vi "flashV4.vi"() -> ()   [LabVIEW 2017]
panel:
  out "error out 2":errorcluster={"status"=TRUE, "code"=56, "source"="UDP Read in UDP.vi->flash.vi"}
  out "error out":errorcluster={"status"=TRUE, "code"=56, "source"="UDP Read in UDP.vi->flash.vi"}
  out "Out 2":u8 format="%.0x"
  out "data out 3":string
  out "data out 2":string
  out "Array":i32[](array[numeric])
  out "String":string
  in  "error in (no error)":errorcluster
  out "Out":u8 format="%.0x"
  in  "address":string="192.168.10.23"
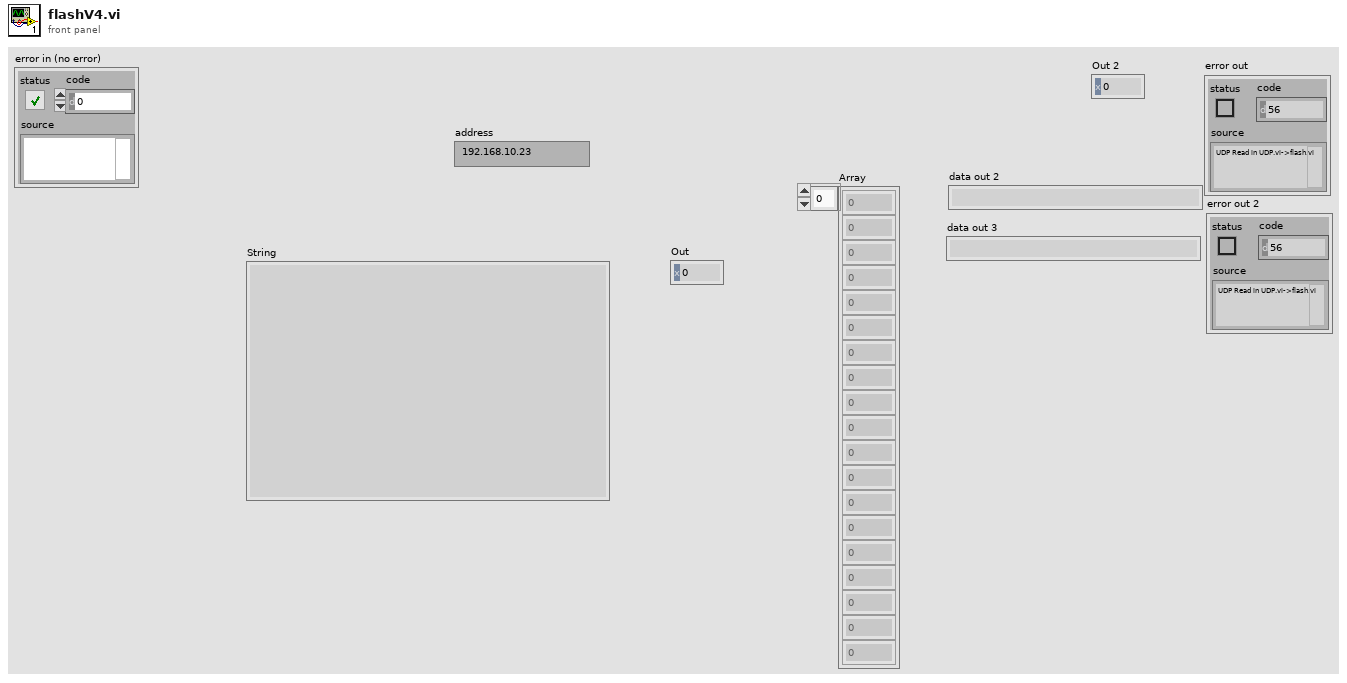
[diagram p1: front panel]
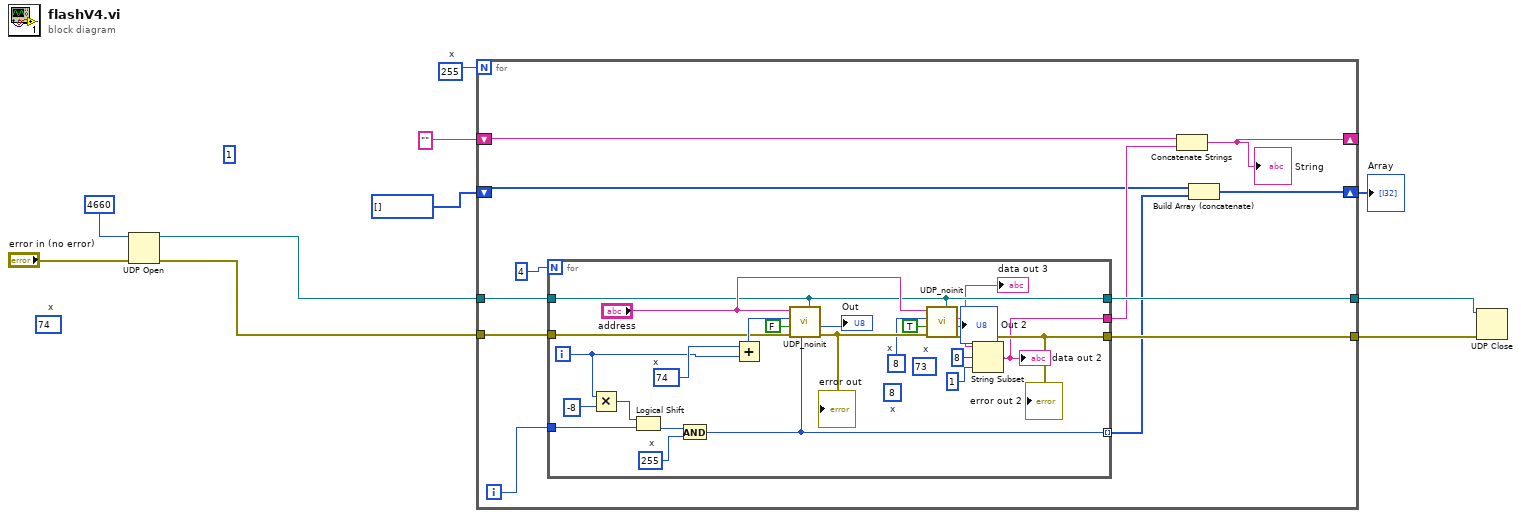
[diagram p0: block diagram]
diagram:
  w5 = u16 255  # x
  (unwired) 1
  (unwired) u16 74  # x
  n1 = UDP Open(8:"error in (no error)", 11:u16 4660 ("UDP port")) -> (port=w8:refnum<k16>, 0:w3:errorcluster)  [unwired: 3 in, 1 out]
  n2 = for {
    N: w5 -> [_]
    tunnel: w8 -> [w20]
    tunnel: [w19] -> w7
    tunnel: [w18] -> w6
    shift-right: [w11] -> _
    shift-left: "" -> [w17]
    tunnel: w3 -> [w15]
    shift-right: [w14] -> w1
    shift-left: u16[] [] -> [w13]
    i -> [w21]
    n3 = for {
      N: 4 -> [_]
      tunnel: w21 -> [w39]
      tunnel: w20 -> [w35]
      tunnel: [w35] -> w19
      tunnel: [w34] -> w18
      tunnel: [w26] -> w16
      tunnel: w15 -> [w32]
      tunnel: [w31] -> w12 mode=indexing
      i -> [w30]
      (unwired) u16 73  # x
      (unwired) u16 8  # x
      w33 = u16 8  # x
      w40 = u16 255  # x
      w43 = u16 74  # x
      n4 = Multiply(x=w30, y=i16 -8) -> (x*y=w38:i32)
      n5 = Logical Shift(y=w38, x=w39) -> (x << y=w41:i32)
      n6 = And(x=w41, y=w40) -> (x .and. y?=w31:i32)
      n7 = Add(x=w43, y=w30) -> (x+y=w42:i32)
      n8 = call "UDP_noinit.vi"("connection ID"=w35, "In"=w31, "error in (no error)"=w32, "Read (TRUE)"=FALSE, "Address"=w42, "IP address"="address") -> ("error out"=w36:errorcluster, "Out"=→"Out":u8)  [unwired: 2 in, 1 out]
      "error out" <- w36
      n9 = call "UDP_noinit.vi"("connection ID"=w35, "error in (no error)"=w36, "Read (TRUE)"=TRUE, "Address"=w33, "IP address"="address") -> ("error out"=w34:errorcluster, "Out"=→"Out 2":u8, "received string"=w25:string)  [unwired: 3 in]
      "data out 3" <- w25
      "error out 2" <- w34
      n10 = String Subset(string=w25, offset (0)=8, length (rest)=1 ("length (rest)")) -> (substring=w26:string)
      "data out 2" <- w26
    }
    n11 = Concatenate Strings(w17, w16) -> (w11:string)
    "String" <- w11
    n12 = Build Array (concatenate)(w13, w12) -> (w14:i32[])
  }
  "Array" <- w1
  n13 = UDP Close(connection ID=w7, 8:w6) -> ()  [unwired: 2 out]
